vi "Teleop.vi"(10 "Match Info":T1={"Autonomous Elapsed Seconds"=0.0, "TeleOp Elapsed Seconds"=0.0, "Disabled Elapsed Seconds"=0.0, "Visited Autonomous"=FALSE, "Visited TeleOp"=FALSE, "Visited Disabled"=FALSE, "Autonomous Settings"={"Autonomous Style"=enum."Independent", "VI Refnum"=refnum}}, 11 "Call Context":T2) -> ()   [LabVIEW 2020]
doc: "This VI is called for each TeleOp packet received from the DS where the robot is not disabled. It is often used to read from the joysticks and update I/O or to update setpoints for timed control loops. It should complete and return within 20 milliseconds or it may miss DS packets."
uses:
  <vilib>/Rock Robotics/WPI/DriverStation/WPI_DriverStationDerivedRobotMode.ctl
  <vilib>/Rock Robotics/WPI/DriverStation/WPI_DriverStationMatch Info.ctl
  <vilib>/Rock Robotics/WPI/Utilities/WPI_GetSetVariantRefNum.vi
  Robot Global Data.vi
  <vilib>/Rock Robotics/Network Tables/NT Write Numeric Array.vi
  <vilib>/Rock Robotics/Network Tables/NT Read Boolean.vi
  <vilib>/Rock Robotics/Network Tables/NT Write Boolean Array.vi
  <vilib>/Rock Robotics/Network Tables/NT Read Number.vi
panel:
  out "Sample Slider 0":dbl(slide) scale=0.0..5.0
  out "Sample Boolean 1":bool
  out "Sample Boolean 0":bool
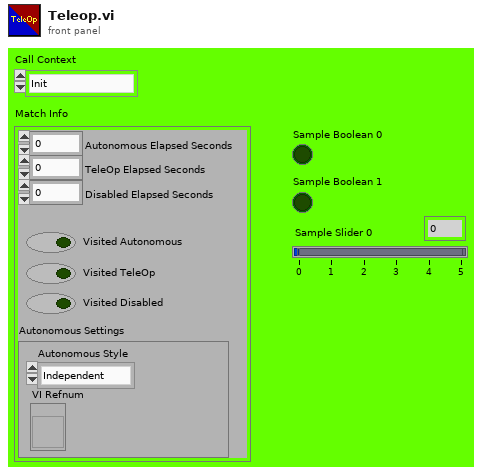
[diagram p1: front panel]
types:
  T1 = typedef "WPI_DriverStationMatch Info.ctl" = cluster{"Autonomous Elapsed Seconds":dbl, "TeleOp Elapsed Seconds":dbl, "Disabled Elapsed Seconds":dbl, "Visited Autonomous":bool, "Visited TeleOp":bool, "Visited Disabled":bool, "Autonomous Settings":cluster{"Autonomous Style":enum16{"Iterative", "Independent"}, "VI Refnum":refnum<vi>}}
  T2 = typedef "WPI_DriverStationDerivedRobotMode.ctl" = enum16{"Init", "Execute", "Stop"}
  T3 = typedef "WPI_JoystickDevRef.ctl" = cluster{"Device":T4}
  T4 = typedef "WPI_JoystickDeviceEnum.ctl" = enum16{"USB 0", "USB 1", "USB 2", "USB 3", "USB 4", "USB 5"}
  T5 = cluster{"Axes[0]":dbl, "Axes[1]":dbl, "Axes[2]":dbl, "Axes[3]":dbl, "Axes[4]":dbl, "Axes[5]":dbl, "Axes[6]":dbl, "Axes[7]":dbl}
  T6 = cluster{"Buttons[0]":bool, "Buttons[1]":bool, "Buttons[2]":bool, "Buttons[3]":bool, "Buttons[4]":bool, "Buttons[5]":bool, "Buttons[6]":bool, "Buttons[7]":bool, "Buttons[8]":bool, "Buttons[9]":bool, "Buttons[10]":bool, "Buttons[11]":bool, "Buttons[12]":bool, "Buttons[13]":bool, "Buttons[14]":bool, "Buttons[15]":bool, "Buttons[16]":bool, "Buttons[17]":bool, "Buttons[18]":bool, "Buttons[19]":bool, "Buttons[20]":bool, "Buttons[21]":bool, "Buttons[22]":bool, "Buttons[23]":bool, "Buttons[24]":bool, "Buttons[25]":bool, "Buttons[26]":bool, "Buttons[27]":bool, "Buttons[28]":bool, "Buttons[29]":bool, "Buttons[30]":bool, "Buttons[31]":bool, "Buttons[32]":bool, "Buttons[33]":bool, "Buttons[34]":bool, "Buttons[35]":bool, "Buttons[36]":bool, "Buttons[37]":bool, "Buttons[38]":bool, "Buttons[39]":bool, "Buttons[40]":bool, "Buttons[41]":bool, "Buttons[42]":bool, "Buttons[43]":bool, "Buttons[44]":bool, "Buttons[45]":bool, "Buttons[46]":bool, "Buttons[47]":bool, "Buttons[48]":bool, "Buttons[49]":bool}
  T7 = cluster{"POVs[0]":i16, "POVs[1]":i16, "POVs[2]":i16, "POVs[3]":i16, "POVs[4]":i16, "POVs[5]":i16, "POVs[6]":i16, "POVs[7]":i16, "POVs[8]":i16}
  T8 = enum16{"Do Nothing", "Cargo", "Low", "High", "Long Shot", "U", "Hook", "Tee", "Eject"}
  T9 = typedef "WPI_RobotDriveDevRef.ctl" = cluster{"DevStatus":errorcluster, "Motors[]":T10[], "Square Inputs":bool, "Max Output":dbl}
  T10 = typedef "WPI_MotorControlDeviceRef.ctl" = cluster{"DeviceStatus":errorcluster, "Type":T11, "PWM":cluster{"PWM Channel":T12, "DeadBand":T13}, "CAN":cluster{"Device Number":u8, "SetOutput VI Ref":variant, "GetOutput VI Ref":variant, "Enable VI Ref":variant, "Disable VI Ref":variant, "Data":variant}, "Invert":bool, "DIO PWM":cluster{"PWM \"Enable\" Channel":T12, "DIOChannel":T14, "PWM Rate":dbl}}
  T11 = typedef "WPI_MotorControlType.ctl" = enum16{"PWM", "CAN", "DIO PWM"}
  T12 = typedef "FPGA_DIOPWMChannel.ctl" = enum8{"PWM 0", "PWM 1", "PWM 2", "PWM 3", "PWM 4", "PWM 5", "PWM 6", "PWM 7", "PWM 8", "PWM 9", "PWM MXP 0", "PWM MXP 1", "PWM MXP 2", "PWM MXP 3", "PWM MXP 4", "PWM MXP 5", "PWM MXP 6", "PWM MXP 7", "PWM MXP 8", "PWM MXP 9", "Invalid"}
  T13 = typedef "WPI_PWMDeadband.ctl" = cluster{"Name":string, "maxPositivePwm":i32, "minPositivePwm":i32, "centerPwm":i32, "maxNegativePwm":i32, "minNegativePwm":i32, "angularRange":u16}
  T14 = typedef "FPGA_DIOChannel.ctl" = enum8{"DIO 0", "DIO 1", "DIO 2", "DIO 3", "DIO 4", "DIO 5", "DIO 6", "DIO 7", "DIO 8", "DIO 9", "DIO MXP 0", "DIO MXP 1", "DIO MXP 2", "DIO MXP 3", "DIO MXP 4", "DIO MXP 5", "DIO MXP 6", "DIO MXP 7", "DIO MXP 8", "DIO MXP 9", "DIO MXP 10", "DIO MXP 11", "DIO MXP 12", "DIO MXP 13", "DIO MXP 14", "DIO MXP 15", "SPI Port CS1", "SPI Port CS2", "SPI Port CS3", "SPI Port MISO", "SPI Port MOSI", "Invalid"}
  T15 = cluster{"A1":dbl, "A2":dbl, "A3":dbl, "A4":dbl, "A5":dbl, "A6":dbl, "A7":dbl, "A8":dbl}
  T16 = cluster{"1":bool, "2":bool, "3":bool, "4":bool, "5":bool, "6":bool, "7":bool, "8":bool, "9":bool, "10":bool, "11":bool, "12":bool, "13":bool, "14":bool, "15":bool, "16":bool, "17":bool, "18":bool, "19":bool, "20":bool, "21":bool, "22":bool, "23":bool, "24":bool, "25":bool, "26":bool, "27":bool, "28":bool, "29":bool, "30":bool, "31":bool, "32":bool, "33":bool, "34":bool, "35":bool, "36":bool, "37":bool, "38":bool, "39":bool, "40":bool, "41":bool, "42":bool, "43":bool, "44":bool, "45":bool, "46":bool, "47":bool, "48":bool, "49":bool, "50":bool}
  T17 = enum16{"Do Nothing", "Cargo", "Low", "High", "Long Shot", "U", "Hook", "Tee"}
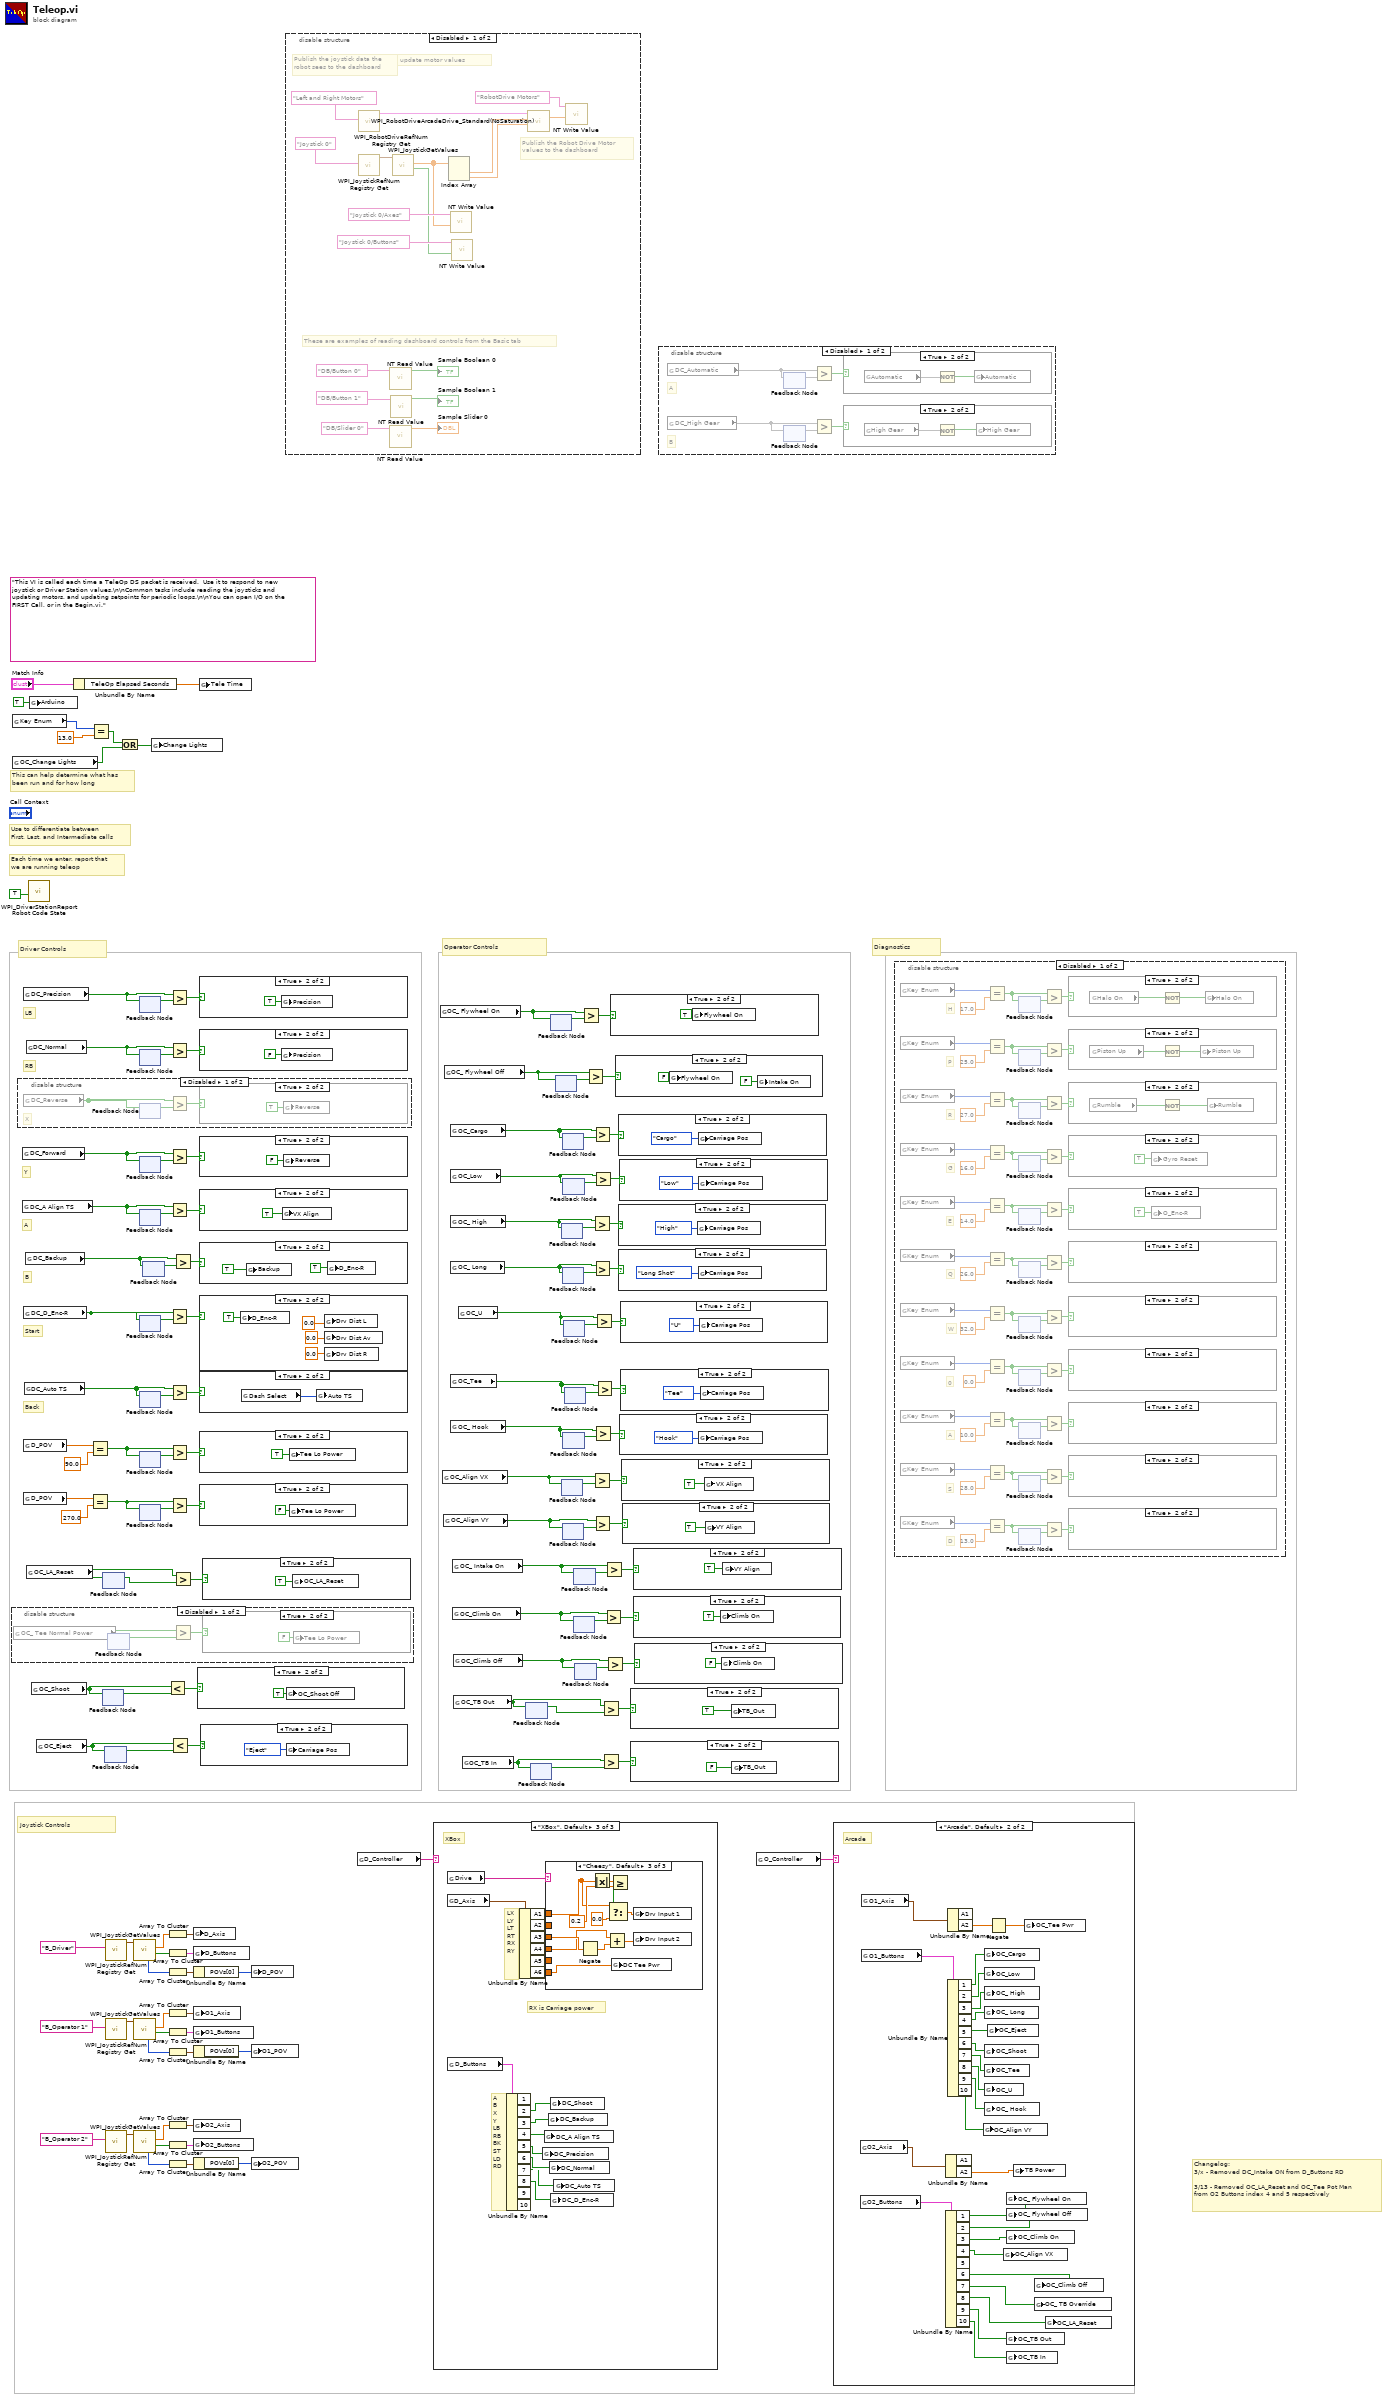
[diagram p0: block diagram]
diagram:
  (unwired) "This VI is called each time a TeleOp DS packet is received.  Use it to respond to new joystick or Driver Station values.\n\nCommon tasks include reading the joysticks and updating motors, and updating setpoints for periodic loops.\n\nYou can open I/O on the FIRST Call, or in the Begin.vi."
  # "Changelog:\n3/x - Removed DC_Intake ON from D_Buttons RD\n\n3/13 - Removed OC_LA_Reset and OC_Tee Pot Man\nfrom O2 Buttons index 4 and 5 respectively"
  # "RB"
  # "Back"
  # "B"
  # "Start"
  # "Y"
  # "A"
  # "LB"
  # "Joystick Controls"
  # "Diagnostics"
  # "Operator Controls"
  # "Driver Controls"
  # "Each time we enter, report that\nwe are running teleop"
  # "Use to differentiate between\nFirst, Last, and Intermediate calls"
  # "This can help determine what has\nbeen run and for how long"
  n1 = disable-structure shown="Disabled" {
    frame Disabled {
      n2 = global read "Robot Global Data.vi" "OC_ Tee Normal Power"() -> (w127:bool)
      n3 = feedback #1() -> (w128:bool)  [unwired: 1 in]
      n4 = feedback-in #1(w127) -> ()
      n5 = Greater?(x=w127, y=w128) -> (0:w129:bool)
      n6 = case shown="True" w129 {
        frame False {
        }
        frame True {
          n7 = global write "Robot Global Data.vi" "Tee Lo Power"(FALSE ("High Gear")) -> ()
        }
      }
    }
    frame Enabled {
    }
  }
  n8 = global read "Robot Global Data.vi" "Key Enum"() -> (w14:i16)
  n9 = global read "Robot Global Data.vi" "OC_Change Lights"() -> (w11:bool)
  n10 = disable-structure shown="Disabled" {
    frame Disabled {
      # "X"
      n11 = global read "Robot Global Data.vi" "DC_Reverse"() -> (w131:bool)
      n12 = feedback #2() -> (w132:bool)  [unwired: 1 in]
      n13 = feedback-in #2(w131) -> ()
      n14 = Greater?(x=w131, y=w132) -> (0:w133:bool)
      n15 = case shown="True" w133 {
        frame False {
        }
        frame True {
          n16 = global write "Robot Global Data.vi" "Reverse"(TRUE ("Reverse")) -> ()
        }
      }
    }
    frame Enabled {
    }
  }
  n17 = global read "Robot Global Data.vi" "DC_Forward"() -> (w87:bool)
  n18 = global read "Robot Global Data.vi" "DC_A Align TS"() -> (w78:bool)
  n19 = global read "Robot Global Data.vi" "DC_Precision"() -> (w86:bool)
  n20 = global read "Robot Global Data.vi" "DC_D_Enc-R"() -> (w84:bool)
  n21 = global read "Robot Global Data.vi" "D_POV"() -> (w96:dbl)
  n22 = global read "Robot Global Data.vi" "D_POV"() -> (w80:dbl)
  n23 = global read "Robot Global Data.vi" "DC_Auto TS"() -> (w69:bool)
  n24 = global read "Robot Global Data.vi" "DC_Backup"() -> (w73:bool)
  n25 = global read "Robot Global Data.vi" "DC_Normal"() -> (w64:bool)
  n26 = global read "Robot Global Data.vi" "OC_LA_Reset"() -> (w30:bool)
  n27 = call <vilib>:"WPI_DriverStationReport Robot Code State.vi"("TeleOp"=TRUE ("Autonomous")) -> ()  [unwired: 10 in, 1 out]
  n28 = global write "Robot Global Data.vi" "Arduino"(TRUE ("Arduino")) -> ()
  n29 = global read "Robot Global Data.vi" "OC_Shoot"() -> (w6:bool)
  n30 = global read "Robot Global Data.vi" "OC_Eject"() -> (w3:bool)
  n31 = Unbundle By Name("Match Info") -> ("TeleOp Elapsed Seconds"=w16:dbl)
  n32 = Equal?(x=w96, y=90.0) -> (x = y?=w85:bool)
  n33 = Equal?(x=w80, y=270.0) -> (x = y?=w83:bool)
  n34 = Equal?(x=w14, y=13.0) -> (x = y?=w12:bool)
  n35 = feedback #3() -> (w5:bool)  [unwired: 1 in]
  n36 = feedback-in #3(w6) -> ()
  n37 = feedback #4() -> (w29:bool)  [unwired: 1 in]
  n38 = feedback-in #4(w30) -> ()
  n39 = feedback #5() -> (w2:bool)  [unwired: 1 in]
  n40 = feedback-in #5(w3) -> ()
  n41 = call <vilib>:"WPI_JoystickRefNum Registry Get.vi"("refnum name"="B_Driver") -> ("JoystickDevRef"=w124:T3)  [unwired: 9 in, 1 out]
  n42 = call <vilib>:"WPI_JoystickRefNum Registry Get.vi"("refnum name"="B_Operator 1") -> ("JoystickDevRef"=w110:T3)  [unwired: 9 in, 1 out]
  n43 = call <vilib>:"WPI_JoystickRefNum Registry Get.vi"("refnum name"="B_Operator 2") -> ("JoystickDevRef"=w107:T3)  [unwired: 9 in, 1 out]
  n44 = Or(x=w12, y=w11) -> (x .or. y?=w10:bool)
  n45 = call <vilib>:"WPI_JoystickGetValues.vi"("JoystickDevRef"=w124) -> ("Buttons"=w122:bool[], "Axes"=w121:dbl[], "POVs"=w120:i16[])  [unwired: 6 in, 2 out]
  n46 = call <vilib>:"WPI_JoystickGetValues.vi"("JoystickDevRef"=w110) -> ("Buttons"=w112:bool[], "Axes"=w113:dbl[], "POVs"=w114:i16[])  [unwired: 6 in, 2 out]
  n47 = call <vilib>:"WPI_JoystickGetValues.vi"("JoystickDevRef"=w107) -> ("Buttons"=w105:bool[], "Axes"=w104:dbl[], "POVs"=w103:i16[])  [unwired: 6 in, 2 out]
  n48 = feedback #6() -> (w93:bool)  [unwired: 1 in]
  n49 = feedback-in #6(w86) -> ()
  n50 = feedback #7() -> (w66:bool)  [unwired: 1 in]
  n51 = feedback-in #7(w64) -> ()
  n52 = feedback #8() -> (w94:bool)  [unwired: 1 in]
  n53 = feedback-in #8(w87) -> ()
  n54 = feedback #9() -> (w76:bool)  [unwired: 1 in]
  n55 = feedback-in #9(w78) -> ()
  n56 = feedback #10() -> (w91:bool)  [unwired: 1 in]
  n57 = feedback-in #10(w84) -> ()
  n58 = feedback #11() -> (w67:bool)  [unwired: 1 in]
  n59 = feedback-in #11(w69) -> ()
  n60 = feedback #12() -> (w89:bool)  [unwired: 1 in]
  n61 = feedback-in #12(w85) -> ()
  n62 = feedback #13() -> (w81:bool)  [unwired: 1 in]
  n63 = feedback-in #13(w83) -> ()
  n64 = feedback #14() -> (w72:bool)  [unwired: 1 in]
  n65 = feedback-in #14(w73) -> ()
  n66 = global write "Robot Global Data.vi" "Change Lights"(w10) -> ()
  n67 = Less?(x=w6, y=w5) -> (x < y?=w4:bool)
  n68 = Array To Cluster(array=w121) -> (cluster=w118:T5)
  n69 = Array To Cluster(array=w122) -> (cluster=w117:T6)
  n70 = Array To Cluster(array=w120) -> (cluster=w119:T7)
  n71 = Array To Cluster(array=w113) -> (cluster=w109:T5)
  n72 = Array To Cluster(array=w112) -> (cluster=w116:T6)
  n73 = Array To Cluster(array=w114) -> (cluster=w115:T7)
  n74 = Array To Cluster(array=w104) -> (cluster=w108:T5)
  n75 = Array To Cluster(array=w105) -> (cluster=w101:T6)
  n76 = Array To Cluster(array=w103) -> (cluster=w102:T7)
  n77 = Greater?(x=w86, y=w93) -> (0:w92:bool)
  n78 = Greater?(x=w64, y=w66) -> (0:w65:bool)
  n79 = Greater?(x=w87, y=w94) -> (0:w95:bool)
  n80 = Greater?(x=w78, y=w76) -> (0:w77:bool)
  n81 = Greater?(x=w84, y=w91) -> (0:w90:bool)
  n82 = Greater?(x=w69, y=w67) -> (0:w68:bool)
  n83 = Greater?(x=w85, y=w89) -> (0:w88:bool)
  n84 = Greater?(x=w83, y=w81) -> (0:w82:bool)
  n85 = Less?(x=w3, y=w2) -> (x < y?=w1:bool)
  n86 = Greater?(x=w73, y=w72) -> (0:w71:bool)
  n87 = Greater?(x=w30, y=w29) -> (0:w31:bool)
  n88 = global write "Robot Global Data.vi" "D_Axis"(w118) -> ()
  n89 = global write "Robot Global Data.vi" "D_Buttons"(w117) -> ()
  n90 = Unbundle By Name(w119) -> ("POVs[0]"=w100:i16)
  n91 = global write "Robot Global Data.vi" "O1_Axis"(w109) -> ()
  n92 = global write "Robot Global Data.vi" "O1_Buttons"(w116) -> ()
  n93 = Unbundle By Name(w115) -> ("POVs[0]"=w99:i16)
  n94 = global write "Robot Global Data.vi" "O2_Axis"(w108) -> ()
  n95 = global write "Robot Global Data.vi" "O2_Buttons"(w101) -> ()
  n96 = Unbundle By Name(w102) -> ("POVs[0]"=w98:i16)
  n97 = case shown="True" w4 {
    frame False {
    }
    frame True {
      n98 = global write "Robot Global Data.vi" "OC_Shoot Off"(TRUE ("High Gear")) -> ()
    }
  }
  n99 = global write "Robot Global Data.vi" "Tele Time"(w16) -> ()
  n100 = case shown="True" w92 {
    frame False {
    }
    frame True {
      n101 = global write "Robot Global Data.vi" "Precision"(TRUE ("Precision")) -> ()
    }
  }
  n102 = case shown="True" w65 {
    frame False {
    }
    frame True {
      n103 = global write "Robot Global Data.vi" "Precision"(FALSE ("Precision")) -> ()
    }
  }
  n104 = case shown="True" w95 {
    frame False {
    }
    frame True {
      n105 = global write "Robot Global Data.vi" "Reverse"(FALSE ("Reverse")) -> ()
    }
  }
  n106 = case shown="True" w77 {
    frame False {
    }
    frame True {
      n107 = global write "Robot Global Data.vi" "VX Align"(TRUE ("Auto Align TS")) -> ()
    }
  }
  n108 = case shown="True" w71 {
    frame False {
    }
    frame True {
      n109 = global write "Robot Global Data.vi" "Backup"(TRUE ("DC_Backup")) -> ()
      n110 = global write "Robot Global Data.vi" "D_Enc-R"(TRUE ("High Gear")) -> ()
    }
  }
  n111 = case shown="True" w90 {
    frame False {
    }
    frame True {
      n112 = global write "Robot Global Data.vi" "D_Enc-R"(TRUE ("High Gear")) -> ()
      n113 = global write "Robot Global Data.vi" "Drv Dist L"(0.0 ("Drv Dist L")) -> ()
      n114 = global write "Robot Global Data.vi" "Drv Dist Av"(0.0 ("Drv Dist Av")) -> ()
      n115 = global write "Robot Global Data.vi" "Drv Dist R"(0.0 ("Drv Dist R")) -> ()
    }
  }
  n116 = case shown="True" w68 {
    frame False {
    }
    frame True {
      n117 = global read "Robot Global Data.vi" "Dash Select"() -> (w146:i8)
      n118 = global write "Robot Global Data.vi" "Auto TS"(w146) -> ()
    }
  }
  n119 = case shown="True" w88 {
    frame False {
    }
    frame True {
      n120 = global write "Robot Global Data.vi" "Tee Lo Power"(TRUE ("High Gear")) -> ()
    }
  }
  n121 = case shown="True" w82 {
    frame False {
    }
    frame True {
      n122 = global write "Robot Global Data.vi" "Tee Lo Power"(FALSE ("High Gear")) -> ()
    }
  }
  n123 = case shown="True" w1 {
    frame False {
    }
    frame True {
      n124 = global write "Robot Global Data.vi" "Carriage Pos"(T8."Eject" ("Carriage Pos")) -> ()
    }
  }
  n125 = case shown="True" w31 {
    frame False {
    }
    frame True {
      n126 = global write "Robot Global Data.vi" "OC_LA_Reset"(TRUE ("High Gear")) -> ()
    }
  }
  n127 = global write "Robot Global Data.vi" "D_POV"(w100) -> ()
  n128 = global write "Robot Global Data.vi" "O1_POV"(w99) -> ()
  n129 = global write "Robot Global Data.vi" "O2_POV"(w98) -> ()
  n130 = disable-structure shown="Disabled" {
    frame Disabled {
      # "These are examples of reading dashboard controls from the Basic tab"
      # "Publish the Robot Drive Motor\nvalues to the dashboard"
      # "Publish the joystick data the\nrobot sees to the dashboard"
      # "Read Joystick X and Y values and update motor values"
      n131 = call <vilib>:"WPI_RobotDriveRefNum Registry Get.vi"("refnum name"="Left and Right Motors") -> ("RobotDriveDevRef"=w167:T9)  [unwired: 1 in, 9 out]
      n132 = call <vilib>:"WPI_JoystickRefNum Registry Get.vi"("refnum name"="Joystick 0") -> ("JoystickDevRef"=w164:T3)  [unwired: 1 in, 9 out]
      n133 = call-poly <vilib>:"NT Read Value.vi"("Name"="DB/Button 0" ("refnum name")) -> ("Boolean"=→"Sample Boolean 0":bool)  [unwired: 9 in, 1 out]
      n134 = call-poly <vilib>:"NT Read Value.vi"("Name"="DB/Slider 0" ("refnum name")) -> ("Numeric"=→"Sample Slider 0":dbl)  [unwired: 9 in, 1 out]
      n135 = call-poly <vilib>:"NT Read Value.vi"("Name"="DB/Button 1" ("refnum name")) -> ("Boolean"=→"Sample Boolean 1":bool)  [unwired: 9 in, 1 out]
      n136 = call <vilib>:"WPI_JoystickGetValues.vi"("JoystickDevRef"=w164) -> ("Buttons"=w159:bool[], "Axes"=w160:dbl[])  [unwired: 6 in, 3 out]
      n137 = Index Array(array=w160) -> (element #1=w166:dbl, element #2=w163:dbl)  [unwired: 2 in]
      n138 = call-poly <vilib>:"NT Write Value.vi"("Numeric Array"=w160, "Name"="Joystick 0/Axes") -> ()  [unwired: 9 in, 1 out]
      n139 = call-poly <vilib>:"NT Write Value.vi"("Boolean Array"=w159, "Name"="Joystick 0/Buttons") -> ()  [unwired: 9 in, 1 out]
      n140 = call <vilib>:"WPI_RobotDriveArcadeDrive_Standard(NoSaturation).vi"("Y axis value"=w163, "X axis value"=w166, "RobotDriveDevRef"=w167) -> ("Motor Values"=w152:dbl[])  [unwired: 1 in, 7 out]
      n141 = call-poly <vilib>:"NT Write Value.vi"("Numeric Array"=w152, "Name"="RobotDrive Motors") -> ()  [unwired: 9 in, 1 out]
    }
    frame Enabled {
    }
  }
  n142 = global read "Robot Global Data.vi" "D_Controller"() -> (w75:string)
  n143 = case shown="\"XBox\", Default" w75 {
    frame "Sticks" {
    }
    frame "Steering" {
    }
    frame "XBox", Default {
      # "RX is Carriage power"
      # "LX\nLY\nLT\nRT\nRX\nRY"
      # "A\nB\nX\nY\nLB\nRB\nBK\nST\nLD\nRD"
      # "XBox"
      n144 = global read "Robot Global Data.vi" "D_Axis"() -> (w184:T15)
      n145 = global read "Robot Global Data.vi" "Drive"() -> (w183:string)
      n146 = global read "Robot Global Data.vi" "D_Buttons"() -> (w177:T16)
      n147 = Unbundle By Name(w177) -> ("2"=w169:bool, "3"=w170:bool, "4"=w171:bool, "5"=w176:bool, "6"=w175:bool, "7"=w173:bool, "8"=w174:bool)  [unwired: 3 out]
      n148 = Unbundle By Name(w184) -> ("A1"=w182:dbl, "A2"=w179:dbl, "A3"=w181:dbl, "A4"=w180:dbl, "A5"=w172:dbl, "A6"=w178:dbl)
      n149 = global write "Robot Global Data.vi" "DC_Precision"(w176) -> ()
      n150 = global write "Robot Global Data.vi" "DC_A Align TS"(w171) -> ()
      n151 = case shown="\"Cheesy\", Default" w183 {
        tunnel: w182 -> [_ w188 w192]
        tunnel: w181 -> [_ _ w199]
        tunnel: w180 -> [_ _ w198]
        tunnel: w179 -> [w186 w187 _]
        tunnel: w178 -> [w185 _ w191]
        tunnel: w172 -> [_ _ _]
        frame "Tank" {
          n152 = global write "Robot Global Data.vi" "Drv Input 1"(w186) -> ()
          n153 = global write "Robot Global Data.vi" "Drv Input 2"(w185) -> ()
        }
        frame "Arcade" {
          n154 = Multiply(x=w187, y=-1.0) -> (x*y=w189:dbl)
          n155 = global write "Robot Global Data.vi" "Drv Input 1"(w188) -> ()
          n156 = global write "Robot Global Data.vi" "Drv Input 2"(w189) -> ()
        }
        frame "Cheesy", Default {
          n157 = Negate(x=w199) -> (-x=w201:dbl)
          n158 = Absolute Value(x=w192) -> (abs(x)=w193:dbl)
          n159 = Add(x=w198, y=w201) -> (x+y=w200:dbl)
          n160 = Greater Or Equal?(x=w193, y=0.2) -> (x >= y?=w195:bool)
          n161 = Select(t=w192, s=w195, f=0.0) -> (s? t:f=w197:dbl)
          n162 = global write "Robot Global Data.vi" "DC Tee Pwr"(w191) -> ()
          n163 = global write "Robot Global Data.vi" "Drv Input 1"(w197) -> ()
          n164 = global write "Robot Global Data.vi" "Drv Input 2"(w200) -> ()
        }
      }
      n165 = global write "Robot Global Data.vi" "DC_Backup"(w170) -> ()
      n166 = global write "Robot Global Data.vi" "DC_Normal"(w175) -> ()
      n167 = global write "Robot Global Data.vi" "DC_Shoot"(w169) -> ()
      n168 = global write "Robot Global Data.vi" "DC_D_Enc-R"(w174) -> ()
      n169 = global write "Robot Global Data.vi" "DC_Auto TS"(w173) -> ()
    }
  }
  n170 = global read "Robot Global Data.vi" "OC_ Flywheel On"() -> (w20:bool)
  n171 = global read "Robot Global Data.vi" "OC_Align VX"() -> (w41:bool)
  n172 = global read "Robot Global Data.vi" "OC_Align VY"() -> (w7:bool)
  n173 = global read "Robot Global Data.vi" "OC_ Flywheel Off"() -> (w19:bool)
  n174 = global read "Robot Global Data.vi" "OC_Cargo"() -> (w62:bool)
  n175 = global read "Robot Global Data.vi" "OC_Low"() -> (w59:bool)
  n176 = global read "Robot Global Data.vi" "OC_ High"() -> (w56:bool)
  n177 = global read "Robot Global Data.vi" "OC_ Long"() -> (w53:bool)
  n178 = global read "Robot Global Data.vi" "OC_Tee"() -> (w47:bool)
  n179 = global read "Robot Global Data.vi" "OC_ Hook"() -> (w44:bool)
  n180 = global read "Robot Global Data.vi" "OC_ Intake On"() -> (w40:bool)
  n181 = global read "Robot Global Data.vi" "OC_Climb On"() -> (w35:bool)
  n182 = global read "Robot Global Data.vi" "OC_Climb Off"() -> (w34:bool)
  n183 = global read "Robot Global Data.vi" "OC_TB Out"() -> (w27:bool)
  n184 = global read "Robot Global Data.vi" "OC_U"() -> (w50:bool)
  n185 = global read "Robot Global Data.vi" "OC_TB In"() -> (w26:bool)
  n186 = feedback #15() -> (w28:bool)  [unwired: 1 in]
  n187 = feedback-in #15(w27) -> ()
  n188 = feedback #16() -> (w25:bool)  [unwired: 1 in]
  n189 = feedback-in #16(w26) -> ()
  n190 = feedback #17() -> (w22:bool)  [unwired: 1 in]
  n191 = feedback-in #17(w20) -> ()
  n192 = feedback #18() -> (w17:bool)  [unwired: 1 in]
  n193 = feedback-in #18(w19) -> ()
  n194 = feedback #19() -> (w57:bool)  [unwired: 1 in]
  n195 = feedback-in #19(w56) -> ()
  n196 = feedback #20() -> (w43:bool)  [unwired: 1 in]
  n197 = feedback-in #20(w41) -> ()
  n198 = feedback #21() -> (w63:bool)  [unwired: 1 in]
  n199 = feedback-in #21(w62) -> ()
  n200 = feedback #22() -> (w54:bool)  [unwired: 1 in]
  n201 = feedback-in #22(w53) -> ()
  n202 = feedback #23() -> (w9:bool)  [unwired: 1 in]
  n203 = feedback-in #23(w7) -> ()
  n204 = feedback #24() -> (w60:bool)  [unwired: 1 in]
  n205 = feedback-in #24(w59) -> ()
  n206 = feedback #25() -> (w45:bool)  [unwired: 1 in]
  n207 = feedback-in #25(w44) -> ()
  n208 = feedback #26() -> (w51:bool)  [unwired: 1 in]
  n209 = feedback-in #26(w50) -> ()
  n210 = feedback #27() -> (w48:bool)  [unwired: 1 in]
  n211 = feedback-in #27(w47) -> ()
  n212 = feedback #28() -> (w37:bool)  [unwired: 1 in]
  n213 = feedback-in #28(w35) -> ()
  n214 = feedback #29() -> (w38:bool)  [unwired: 1 in]
  n215 = feedback-in #29(w40) -> ()
  n216 = feedback #30() -> (w32:bool)  [unwired: 1 in]
  n217 = feedback-in #30(w34) -> ()
  n218 = Greater?(x=w20, y=w22) -> (0:w21:bool)
  n219 = Greater?(x=w19, y=w17) -> (0:w18:bool)
  n220 = Greater?(x=w56, y=w57) -> (0:w58:bool)
  n221 = Greater?(x=w41, y=w43) -> (0:w42:bool)
  n222 = Greater?(x=w62, y=w63) -> (0:w70:bool)
  n223 = Greater?(x=w53, y=w54) -> (0:w55:bool)
  n224 = Greater?(x=w7, y=w9) -> (0:w8:bool)
  n225 = Greater?(x=w59, y=w60) -> (0:w61:bool)
  n226 = Greater?(x=w44, y=w45) -> (0:w46:bool)
  n227 = Greater?(x=w50, y=w51) -> (0:w52:bool)
  n228 = Greater?(x=w47, y=w48) -> (0:w49:bool)
  n229 = Greater?(x=w27, y=w28) -> (0:w24:bool)
  n230 = Greater?(x=w26, y=w25) -> (0:w23:bool)
  n231 = Greater?(x=w35, y=w37) -> (0:w36:bool)
  n232 = Greater?(x=w40, y=w38) -> (0:w39:bool)
  n233 = Greater?(x=w34, y=w32) -> (0:w33:bool)
  n234 = case shown="True" w21 {
    frame False {
    }
    frame True {
      n235 = global write "Robot Global Data.vi" "Flywheel On"(TRUE ("Intake On")) -> ()
    }
  }
  n236 = case shown="True" w18 {
    frame False {
    }
    frame True {
      n237 = global write "Robot Global Data.vi" "Flywheel On"(FALSE ("Intake On")) -> ()
      n238 = global write "Robot Global Data.vi" "Intake On"(FALSE ("Intake On")) -> ()
    }
  }
  n239 = case shown="True" w58 {
    frame False {
    }
    frame True {
      n240 = global write "Robot Global Data.vi" "Carriage Pos"(T17."High" ("Carriage Pos")) -> ()
    }
  }
  n241 = case shown="True" w70 {
    frame False {
    }
    frame True {
      n242 = global write "Robot Global Data.vi" "Carriage Pos"(T17."Cargo" ("Carriage Pos")) -> ()
    }
  }
  n243 = case shown="True" w55 {
    frame False {
    }
    frame True {
      n244 = global write "Robot Global Data.vi" "Carriage Pos"(T17."Long Shot" ("Carriage Pos")) -> ()
    }
  }
  n245 = case shown="True" w61 {
    frame False {
    }
    frame True {
      n246 = global write "Robot Global Data.vi" "Carriage Pos"(T17."Low" ("Carriage Pos")) -> ()
    }
  }
  n247 = case shown="True" w46 {
    frame False {
    }
    frame True {
      n248 = global write "Robot Global Data.vi" "Carriage Pos"(T17."Hook" ("Carriage Pos")) -> ()
    }
  }
  n249 = case shown="True" w52 {
    frame False {
    }
    frame True {
      n250 = global write "Robot Global Data.vi" "Carriage Pos"(T17."U" ("Carriage Pos")) -> ()
    }
  }
  n251 = case shown="True" w49 {
    frame False {
    }
    frame True {
      n252 = global write "Robot Global Data.vi" "Carriage Pos"(T17."Tee" ("Carriage Pos")) -> ()
    }
  }
  n253 = case shown="True" w42 {
    frame False {
    }
    frame True {
      n254 = global write "Robot Global Data.vi" "VX Align"(TRUE ("Auto Align TS")) -> ()
    }
  }
  n255 = case shown="True" w8 {
    frame False {
    }
    frame True {
      n256 = global write "Robot Global Data.vi" "VY Align"(TRUE ("Auto Align TS")) -> ()
    }
  }
  n257 = case shown="True" w24 {
    frame False {
    }
    frame True {
      n258 = global write "Robot Global Data.vi" "TB_Out"(TRUE ("High Gear")) -> ()
    }
  }
  n259 = case shown="True" w23 {
    frame False {
    }
    frame True {
      n260 = global write "Robot Global Data.vi" "TB_Out"(FALSE ("High Gear")) -> ()
    }
  }
  n261 = case shown="True" w36 {
    frame False {
    }
    frame True {
      n262 = global write "Robot Global Data.vi" "Climb On"(TRUE ("Intake On")) -> ()
    }
  }
  n263 = case shown="True" w39 {
    frame False {
    }
    frame True {
      n264 = global write "Robot Global Data.vi" "VY Align"(TRUE ("Intake On")) -> ()
    }
  }
  n265 = case shown="True" w33 {
    frame False {
    }
    frame True {
      n266 = global write "Robot Global Data.vi" "Climb On"(FALSE ("Intake On")) -> ()
    }
  }
  n267 = disable-structure shown="Disabled" {
    frame Disabled {
      # "A"
      # "B"
      n268 = global read "Robot Global Data.vi" "DC_Automatic"() -> (w224)
      n269 = global read "Robot Global Data.vi" "DC_High Gear"() -> (w223)
      n270 = feedback #31() -> (w221)  [unwired: 1 in]
      n271 = feedback-in #31(w224) -> ()
      n272 = feedback #32() -> (w220)  [unwired: 1 in]
      n273 = feedback-in #32(w223) -> ()
      n274 = Greater?(x=w224, y=w221) -> (0:w222:bool)
      n275 = Greater?(x=w223, y=w220) -> (0:w219:bool)
      n276 = case shown="True" w222 {
        frame False {
        }
        frame True {
          n277 = global read "Robot Global Data.vi" "Automatic"() -> (w226)
          n278 = Not(x=w226) -> (.not. x?=w225:bool)
          n279 = global write "Robot Global Data.vi" "Automatic"(w225) -> ()
        }
      }
      n280 = case shown="True" w219 {
        frame False {
        }
        frame True {
          n281 = global read "Robot Global Data.vi" "High Gear"() -> (w227)
          n282 = Not(x=w227) -> (.not. x?=w228:bool)
          n283 = global write "Robot Global Data.vi" "High Gear"(w228) -> ()
        }
      }
    }
    frame Enabled {
    }
  }
  n284 = global read "Robot Global Data.vi" "O_Controller"() -> (w74:string)
  n285 = case shown="\"Arcade\", Default" w74 {
    frame "XBox" {
      # "LX\nLY\nLT\nRT\nRX\nRY"
      # "A\nB\nX\nY\nLB\nRB\nBK\nST\nLD\nRD"
      # "XBox"
      n286 = global read "Robot Global Data.vi" "O1_Axis"() -> (w229:T15)
      n287 = global read "Robot Global Data.vi" "O1_Buttons"() -> (w230:T16)
      n288 = Unbundle By Name(w229) -> ()  [unwired: 6 out]
      n289 = Unbundle By Name(w230) -> ()  [unwired: 10 out]
    }
    frame "Arcade", Default {
      # "Arcade"
      n290 = global read "Robot Global Data.vi" "O2_Axis"() -> (w253:T15)
      n291 = global read "Robot Global Data.vi" "O2_Buttons"() -> (w254:T16)
      n292 = global read "Robot Global Data.vi" "O1_Axis"() -> (w256:T15)
      n293 = global read "Robot Global Data.vi" "O1_Buttons"() -> (w255:T16)
      n294 = Unbundle By Name(w253) -> ("A2"=w238:dbl)  [unwired: 1 out]
      n295 = Unbundle By Name(w254) -> ("1"=w237:bool, "2"=w236:bool, "3"=w242:bool, "4"=w234:bool, "6"=w241:bool, "7"=w240:bool, "8"=w239:bool, "9"=w252:bool, "10"=w251:bool)  [unwired: 1 out]
      n296 = Unbundle By Name(w256) -> ("A2"=w231:dbl)  [unwired: 1 out]
      n297 = Unbundle By Name(w255) -> ("1"=w248:bool, "2"=w246:bool, "3"=w245:bool, "4"=w249:bool, "5"=w233:bool, "6"=w250:bool, "7"=w247:bool, "8"=w244:bool, "9"=w243:bool, "10"=w235:bool)
      n298 = global write "Robot Global Data.vi" "OC_Align VY"(w235) -> ()
      n299 = global write "Robot Global Data.vi" "OC_Cargo"(w248) -> ()
      n300 = global write "Robot Global Data.vi" "OC_Low"(w246) -> ()
      n301 = global write "Robot Global Data.vi" "OC_ High"(w245) -> ()
      n302 = global write "Robot Global Data.vi" "OC_ Long"(w249) -> ()
      n303 = global write "Robot Global Data.vi" "OC_Shoot"(w250) -> ()
      n304 = global write "Robot Global Data.vi" "OC_Tee"(w247) -> ()
      n305 = global write "Robot Global Data.vi" "OC_U"(w244) -> ()
      n306 = global write "Robot Global Data.vi" "OC_ Hook"(w243) -> ()
      n307 = Negate(x=w231) -> (-x=w232:dbl)
      n308 = global write "Robot Global Data.vi" "OC_Eject"(w233) -> ()
      n309 = global write "Robot Global Data.vi" "OC_Align VX"(w234) -> ()
      n310 = global write "Robot Global Data.vi" "OC_ Flywheel On"(w237) -> ()
      n311 = global write "Robot Global Data.vi" "OC_ Flywheel Off"(w236) -> ()
      n312 = global write "Robot Global Data.vi" "OC_Climb On"(w242) -> ()
      n313 = global write "Robot Global Data.vi" "OC_TB Out"(w252) -> ()
      n314 = global write "Robot Global Data.vi" "OC_TB In"(w251) -> ()
      n315 = global write "Robot Global Data.vi" "TB Power"(w238) -> ()
      n316 = global write "Robot Global Data.vi" "OC_Tee Pwr"(w232) -> ()
      n317 = global write "Robot Global Data.vi" "OC_ TB Override"(w240) -> ()
      n318 = global write "Robot Global Data.vi" "OC_Climb Off"(w241) -> ()
      n319 = global write "Robot Global Data.vi" "OC_LA_Reset"(w239) -> ()
    }
  }
  n320 = disable-structure shown="Disabled" {
    frame Disabled {
      # "P"
      # "E"
      # "G"
      # "H"
      # "R"
      # "A"
      # "D"
      # "S"
      # "0"
      # "W"
      # "Q"
      n321 = global read "Robot Global Data.vi" "Key Enum"() -> (w276:i16)
      n322 = global read "Robot Global Data.vi" "Key Enum"() -> (w261:i16)
      n323 = global read "Robot Global Data.vi" "Key Enum"() -> (w277:i16)
      n324 = global read "Robot Global Data.vi" "Key Enum"() -> (w266:i16)
      n325 = global read "Robot Global Data.vi" "Key Enum"() -> (w267:i16)
      n326 = global read "Robot Global Data.vi" "Key Enum"() -> (w310:i16)
      n327 = global read "Robot Global Data.vi" "Key Enum"() -> (w309:i16)
      n328 = global read "Robot Global Data.vi" "Key Enum"() -> (w306:i16)
      n329 = global read "Robot Global Data.vi" "Key Enum"() -> (w286:i16)
      n330 = global read "Robot Global Data.vi" "Key Enum"() -> (w304:i16)
      n331 = global read "Robot Global Data.vi" "Key Enum"() -> (w303:i16)
      n332 = Equal?(x=w276, y=17.0) -> (x = y?=w272:bool)
      n333 = Equal?(x=w261, y=25.0) -> (x = y?=w257:bool)
      n334 = Equal?(x=w277, y=27.0) -> (x = y?=w281:bool)
      n335 = Equal?(x=w266, y=16.0) -> (x = y?=w262:bool)
      n336 = Equal?(x=w267, y=14.0) -> (x = y?=w271:bool)
      n337 = Equal?(x=w310, y=26.0) -> (x = y?=w291:bool)
      n338 = Equal?(x=w309, y=32.0) -> (x = y?=w290:bool)
      n339 = Equal?(x=w306, y=0.0) -> (x = y?=w289:bool)
      n340 = Equal?(x=w286, y=10.0) -> (x = y?=w282:bool)
      n341 = Equal?(x=w304, y=28.0) -> (x = y?=w288:bool)
      n342 = Equal?(x=w303, y=13.0) -> (x = y?=w287:bool)
      n343 = feedback #33() -> (w274:bool)  [unwired: 1 in]
      n344 = feedback-in #33(w272) -> ()
      n345 = feedback #34() -> (w259:bool)  [unwired: 1 in]
      n346 = feedback-in #34(w257) -> ()
      n347 = feedback #35() -> (w279:bool)  [unwired: 1 in]
      n348 = feedback-in #35(w281) -> ()
      n349 = feedback #36() -> (w264:bool)  [unwired: 1 in]
      n350 = feedback-in #36(w262) -> ()
      n351 = feedback #37() -> (w269:bool)  [unwired: 1 in]
      n352 = feedback-in #37(w271) -> ()
      n353 = feedback #38() -> (w292:bool)  [unwired: 1 in]
      n354 = feedback-in #38(w291) -> ()
      n355 = feedback #39() -> (w295:bool)  [unwired: 1 in]
      n356 = feedback-in #39(w290) -> ()
      n357 = feedback #40() -> (w296:bool)  [unwired: 1 in]
      n358 = feedback-in #40(w289) -> ()
      n359 = feedback #41() -> (w284:bool)  [unwired: 1 in]
      n360 = feedback-in #41(w282) -> ()
      n361 = feedback #42() -> (w298:bool)  [unwired: 1 in]
      n362 = feedback-in #42(w288) -> ()
      n363 = feedback #43() -> (w301:bool)  [unwired: 1 in]
      n364 = feedback-in #43(w287) -> ()
      n365 = Greater?(x=w272, y=w274) -> (0:w273:bool)
      n366 = Greater?(x=w257, y=w259) -> (0:w258:bool)
      n367 = Greater?(x=w281, y=w279) -> (0:w280:bool)
      n368 = Greater?(x=w262, y=w264) -> (0:w263:bool)
      n369 = Greater?(x=w271, y=w269) -> (0:w270:bool)
      n370 = Greater?(x=w291, y=w292) -> (0:w293:bool)
      n371 = Greater?(x=w290, y=w295) -> (0:w294:bool)
      n372 = Greater?(x=w289, y=w296) -> (0:w297:bool)
      n373 = Greater?(x=w282, y=w284) -> (0:w283:bool)
      n374 = Greater?(x=w288, y=w298) -> (0:w299:bool)
      n375 = Greater?(x=w287, y=w301) -> (0:w300:bool)
      n376 = case shown="True" w273 {
        frame False {
        }
        frame True {
          n377 = global read "Robot Global Data.vi" "Halo On"() -> (w316:bool)
          n378 = Not(x=w316) -> (.not. x?=w317:bool)
          n379 = global write "Robot Global Data.vi" "Halo On"(w317) -> ()
        }
      }
      n380 = case shown="True" w258 {
        frame False {
        }
        frame True {
          n381 = global read "Robot Global Data.vi" "Piston Up"() -> (w312:bool)
          n382 = Not(x=w312) -> (.not. x?=w313:bool)
          n383 = global write "Robot Global Data.vi" "Piston Up"(w313) -> ()
        }
      }
      n384 = case shown="True" w280 {
        frame False {
        }
        frame True {
          n385 = global read "Robot Global Data.vi" "Rumble"() -> (w318:bool)
          n386 = Not(x=w318) -> (.not. x?=w319:bool)
          n387 = global write "Robot Global Data.vi" "Rumble"(w319) -> ()
        }
      }
      n388 = case shown="True" w263 {
        frame False {
        }
        frame True {
          n389 = global write "Robot Global Data.vi" "Gyro Reset"(TRUE ("High Gear")) -> ()
        }
      }
      n390 = case shown="True" w270 {
        frame False {
        }
        frame True {
          n391 = global write "Robot Global Data.vi" "O_Enc-R"(TRUE ("High Gear")) -> ()
        }
      }
      n392 = case shown="True" w293 {
        frame False {
        }
        frame True {
        }
      }
      n393 = case shown="True" w294 {
        frame False {
        }
        frame True {
        }
      }
      n394 = case shown="True" w297 {
        frame False {
        }
        frame True {
        }
      }
      n395 = case shown="True" w283 {
        frame False {
        }
        frame True {
        }
      }
      n396 = case shown="True" w299 {
        frame False {
        }
        frame True {
        }
      }
      n397 = case shown="True" w300 {
        frame False {
        }
        frame True {
        }
      }
    }
    frame Enabled {
    }
  }
